vi "DCPower_CreateOutputArray.vi"(4 "current measurements":dbl[](array[numeric]), 6 "voltage measurements":dbl[](array[numeric]), 7 "Rolling Timer":timestamp, 9 "actual count":i32, 10 "Measure Record dt":dbl, 11 "Initial Time":timestamp) -> (3 "Array":dbl[][](array[numeric]))   [LabVIEW 2019]
uses:
  <vilib>/Analysis/1siggen.llb/Ramp Pattern by Delta.vi
  <vilib>/Analysis/NI_AALBase.lvlib
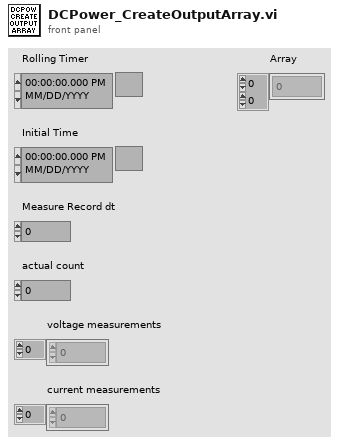
[diagram p1: front panel]
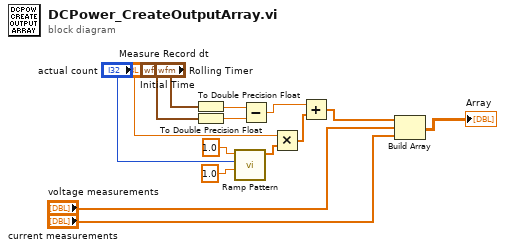
[diagram p0: block diagram]
diagram:
  n1 = To Double Precision Float(number="Rolling Timer") -> (double precision float=w7:dbl)
  n2 = To Double Precision Float(number="Initial Time") -> (double precision float=w8:dbl)
  n3 = call-poly <vilib>:"Ramp Pattern.vi"("start"=1.0, "end"="actual count", "delta"=1.0) -> ("Ramp Pattern"=w2:dbl[])  [unwired: 6 in, 2 out]
  n4 = Subtract(x=w7, y=w8) -> (x-y=w11:dbl)
  n5 = Multiply(x="Measure Record dt", y=w2) -> (x*y=w1:dbl[])
  n6 = Add(x=w11, y=w1) -> (x+y=w15:dbl[])
  n7 = Build Array(w15, "voltage measurements", "current measurements") -> (→"Array":dbl[][])
